vi "ZCAN_InitCAN(USBCANFD).vi"(0 "device_hande":u32, 5 "can_index":u32, 7 "ZCAN_InitCAN_Setting_USBCANFD":T1, 11 "error in (no error)":errorcluster caption="错误输入（无错误）") -> (8 "can_index_handle":u32, 15 "error out":errorcluster caption="错误输出")   [LabVIEW 2018]
doc: "设置CAN卡波特率，工作模式等。\n\n适用的设备：USBCANFD-100U、USBCANFD-200U、USBCANFD-MINI。"
uses:
  zlgcan_demo_CANFDNET_TCP/bin/zlgcan_wrap.dll
  data_type/ZCAN_InitCAN_setting_USBCANFD.ctl
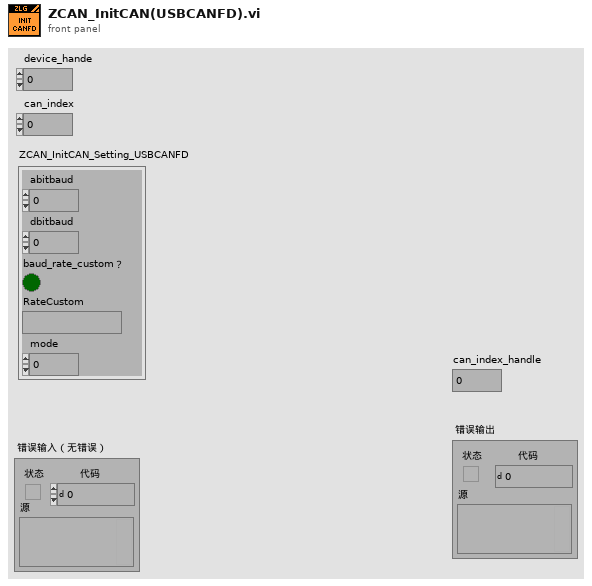
[diagram p1: front panel]
types:
  T1 = typedef "ZCAN_InitCAN_setting_USBCANFD.ctl" = cluster{"abitbaud":u32, "dbitbaud":u32, "baud_rate_custom？":bool, "RateCustom":string, "mode":u8}
  T2 = cluster{"can_type":u32, "can_type":u32, "can_type":u32, "can_type":u32, "can_type":u32, "can_type":u32, u8, "mode":u8, "pad":u16, "reserved":u32}
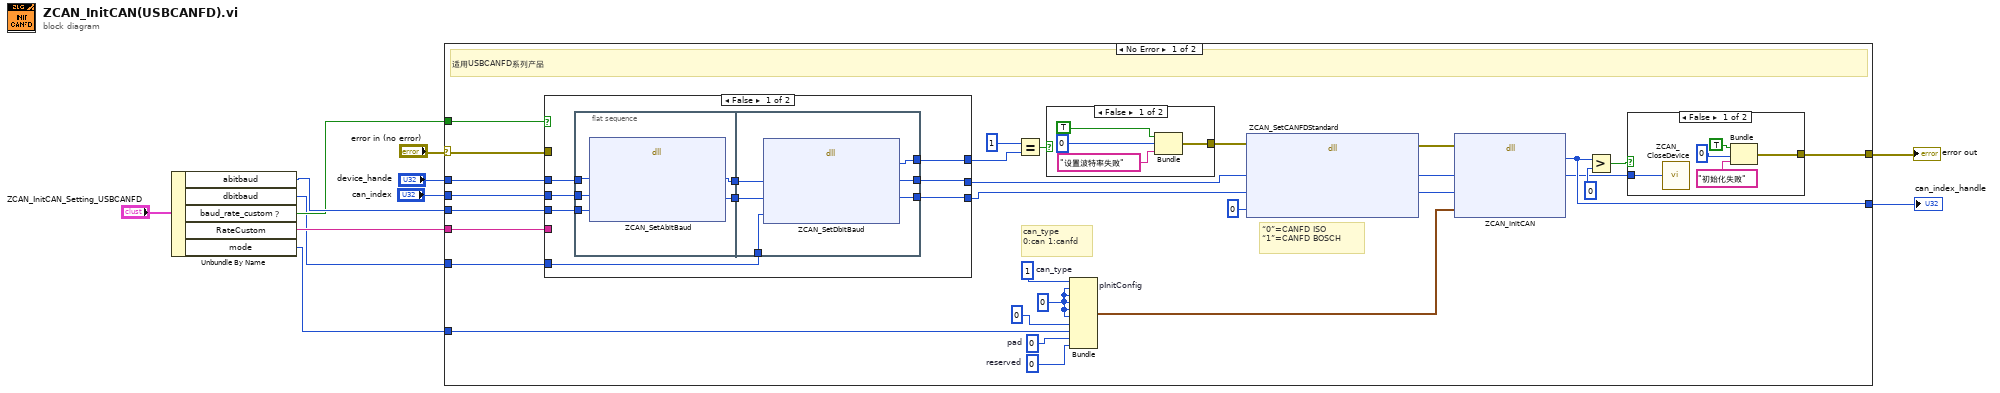
[diagram p0: block diagram]
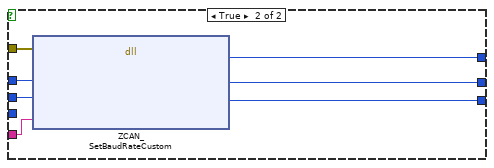
[diagram p4: hidden frame]
diagram:
  n1 = Unbundle By Name("ZCAN_InitCAN_Setting_USBCANFD") -> ("abitbaud"=w5:u32, "dbitbaud"=w1:u32, "baud_rate_custom？"=w4:bool, "RateCustom"=w3:string, "mode"=w2:u8)
  n2 = case shown="No Error" "error in (no error)" {
    selector: "error in (no error)" -> [w35 w77]
    tunnel: [w34 w77] -> w10
    tunnel: w4 -> [w40 _]
    tunnel: "device_hande" -> [w39 _]
    tunnel: "can_index" -> [w38 _]
    tunnel: w5 -> [w37 _]
    tunnel: w3 -> [w36 _]
    tunnel: w2 -> [w19 _]
    tunnel: [w33 _] -> w7
    tunnel: w1 -> [w13 _]
    frame No Error {
      w20 = u32 0  # reserved
      w21 = u16 0  # pad
      w18 = u32 0 ("can_type")
      w22 = u32 1  # can_type
      # "can_type\n0:can 1:canfd"
      # "“0”=CANFD ISO \n“1”=CANFD BOSCH"
      # "适用USBCANFD系列产品"
      n3 = case shown="False" w40 {
        tunnel: [w51 w76] -> w26
        tunnel: [w50 w75] -> w25
        tunnel: [w52 w74] -> w31
        tunnel: w39 -> [w58 w72]
        tunnel: w38 -> [w57 w71]
        tunnel: w37 -> [w56 _]
        tunnel: w36 -> [_ w73]
        tunnel: w35 -> [_ w70]
        tunnel: w13 -> [w53 _]
        frame False {
          n4 = flat-sequence {
            tunnel: w58 -> [w61]
            tunnel: w57 -> [w60]
            tunnel: w56 -> [w59]
            tunnel: [w63] -> w55
            tunnel: [w62] -> w54
            tunnel: w55 -> [w69]
            tunnel: w54 -> [w68]
            tunnel: w53 -> [w67]
            tunnel: [w66] -> w52
            tunnel: [w65] -> w51
            tunnel: [w64] -> w50
            frame #0 {
              n5 = dll-call lib="C:/Users/admin/Desktop/zlgcan_demo_CANFDNET_TCP/bin/zlgcan_wrap.dll" fn="ZCAN_SetAbitBaud" label="设置仲裁域波特率"("device_hande"=w61, "can_index"=w60, "abitbaud"=w59) -> ("device_hande"=w63:u32, "can_index"=w62:u32)  [unwired: 5 in, 2 out]
            }
            frame #1 {
              n6 = dll-call lib="C:/Users/admin/Desktop/zlgcan_demo_CANFDNET_TCP/bin/zlgcan_wrap.dll" fn="ZCAN_SetDbitBaud" label="设置数据域波特率"("device_hande"=w69, "can_index"=w68, "dbitbaud"=w67) -> ("return"=w66:u32, "device_hande"=w65:u32, "can_index"=w64:u32)  [unwired: 4 in, 2 out]
            }
          }
        }
        frame True {
          n7 = dll-call lib="C:/Users/admin/Desktop/zlgcan_demo_CANFDNET_TCP/bin/zlgcan_wrap.dll" fn="ZCAN_SetBaudRateCustom"(error in=w70, "device_handle"=w72, "can_index"=w71, "RateCustom"=w73) -> ("return"=w74:u32, "device_handle"=w76:u32, "can_index"=w75:u32)  [unwired: 3 in, 2 out]
        }
      }
      n8 = Equal?(x=1, y=w31) -> (x = y?=w30:bool)
      n9 = case shown="False" w30 {
        tunnel: [w46 _] -> w27
        frame False {
          n10 = Bundle("status"=TRUE, "code"=0, "消息"="设置波特率失败") -> (w46:cluster{"status":bool, "code":i32, "消息":string})  [unwired: 1 in]
        }
        frame True {
        }
      }
      n11 = Bundle "pInitConfig"("can_type"=w22, "can_type"=w18, "can_type"=w18, "can_type"=w18, "can_type"=w18, "can_type"=w18, u8 0, "mode"=w19, "pad"=w21, "reserved"=w20) -> (w16:T2)  [unwired: 1 in]
      n12 = dll-call lib="C:/Users/admin/Desktop/zlgcan_demo_CANFDNET_TCP/bin/zlgcan_wrap.dll" fn="ZCAN_SetCANFDStandard" ("ZCAN_InitCAN")(error in=w27, "device_handle"=w26, "can_index"=w25, "canfd_standard"=0) -> (error out=w23:errorcluster, "device_handle"=w15:u32, "can_index"=w14:i32)  [unwired: 4 in, 1 out]
      n13 = dll-call lib="C:/Users/admin/Desktop/zlgcan_demo_CANFDNET_TCP/bin/zlgcan_wrap.dll" fn="ZCAN_InitCAN"(error in=w23, "device_handle"=w15, "can_index"=w14, "pInitConfig"=w16) -> ("can_handle"=w33:u32, "device_handle"=w12:u32)  [unwired: 4 in, 2 out]
      n14 = Greater?(x=w33, y=0) -> (0:w28:bool)
      n15 = case shown="False" w28 {
        tunnel: [w42 _] -> w34
        tunnel: w12 -> [w41 _]
        frame False {
          n16 = call "ZCAN_CloseDevice.vi"("device_handle"=w41) -> ()  [unwired: 9 in, 2 out]
          n17 = Bundle("status"=TRUE, "code"=0, "消息"="初始化失败") -> (w42:cluster{"status":bool, "code":i32, "消息":string})  [unwired: 1 in]
        }
        frame True {
        }
      }
    }
    frame Error {
    }
  }
  "error out" <- w10
  "can_index_handle" <- w7
